vi "motor absposi(SubVI).vi"(8 "error in (no error)":errorcluster, 9 "baud rate (9600)":u32=9600, 10 "前進STEP":i32=1000, 11 "VISA Refnum in":refnum<visa-resource-name>) -> (0 "error out":errorcluster, 3 "concatenated string":string="@0X2000,\r\n")   [LabVIEW 2012]
uses:
  <vilib>/Instr/_visa.llb/VISA Configure Serial Port (Instr).vi
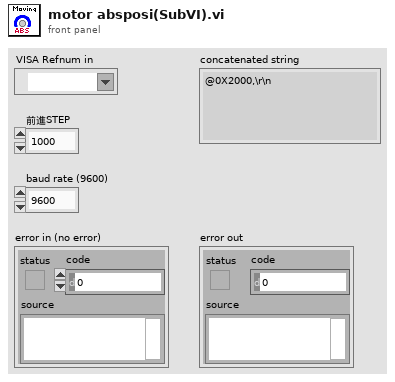
[diagram p1: front panel]
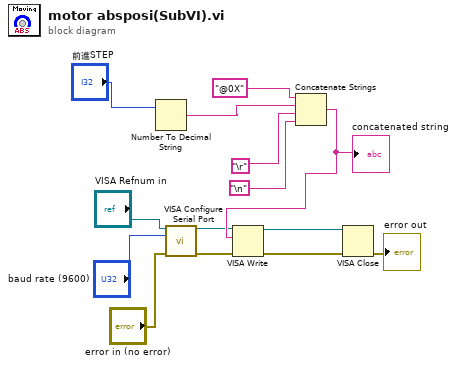
[diagram p0: block diagram]
diagram:
  n1 = Number To Decimal String(number="前進STEP") -> (decimal integer string=w11:string)  [unwired: 1 in]
  n2 = call-poly "VISA Configure Serial Port"("VISA resource name"="VISA Refnum in", "baud rate (9600)"="baud rate (9600)", "error in (no error)"="error in (no error)") -> ("VISA resource name out"=w4:refnum<visa-resource-name>, "error out"=w3:errorcluster)  [unwired: 11 in]
  n3 = Concatenate Strings("@0X", w11, "\r", "\n") -> (w12:string)
  "concatenated string" <- w12
  n4 = VISA Write(VISA resource name=w4, write buffer=w12, error in (no error)=w3) -> (VISA resource name out=w2:refnum<visa-resource-name>, error out=w1:errorcluster)  [unwired: 1 out]
  n5 = VISA Close(VISA resource name=w2, error in (no error)=w1) -> (error out=→"error out":errorcluster)
